vi "Write ASCII Char.vi"(8 "error in (no error)":errorcluster, 9 "Char":string, 11 "LEDMatrix in":refnum<class "LEDAlphaNumeric.lvclass">) -> (0 "error out":errorcluster, 3 "LEDMatrix out":refnum<class "LEDAlphaNumeric.lvclass">)   [LabVIEW 2020, in "CTI-Peripheral.lvlib" / "LEDAlphaNumeric.lvclass"]
uses:
  LEDAlphaNumeric.lvclass
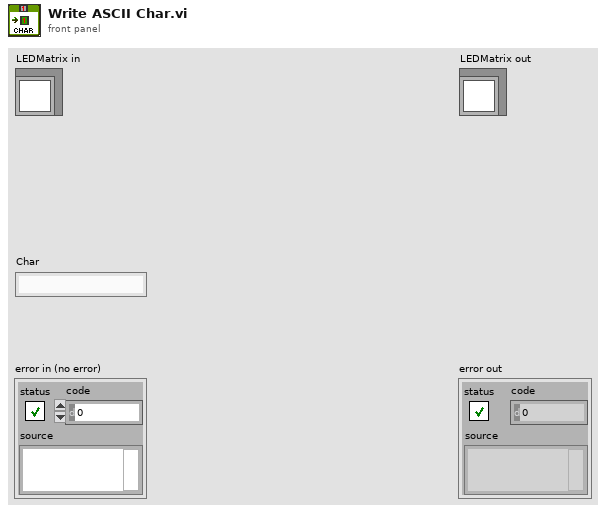
[diagram p1: front panel]
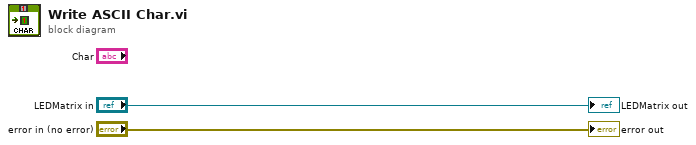
[diagram p0: block diagram]
diagram:
  "error out" <- "error in (no error)"
  "LEDMatrix out" <- "LEDMatrix in"
